vi "Curve Keypair.vi"(7 "path override":path, 8 "error in (no error)":errorcluster, 10 "z85_secret_key_":string, 11 "z85_public_key_":string) -> (0 "error out":errorcluster, 2 "z85_secret_key_ out":string, 3 "z85_public_key_ out":string)   [LabVIEW 2025, in "LibZMQ.lvlib"]
doc: "ZMQ_EXPORT int zmq_curve_keypair (char *z85_public_key_, char *z85_secret_key_);"
uses:
  LibZMQ.lvlib
  errno.vi
  strerror.vi
  <vilib>/Utility/error.llb/Error Cluster From Error Code.vi
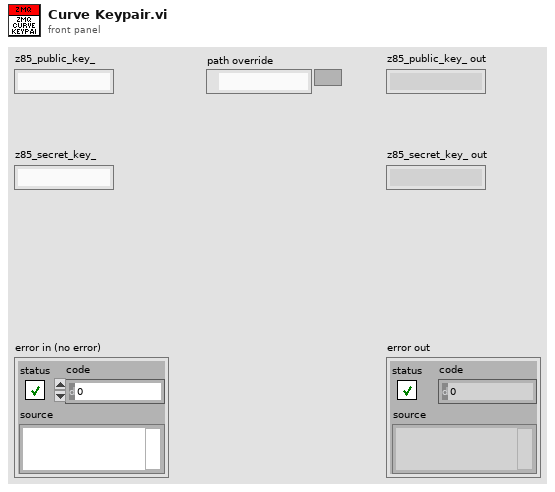
[diagram p1: front panel]
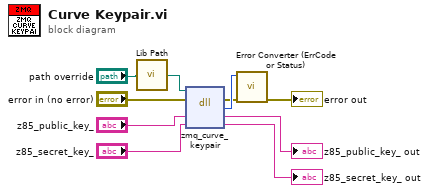
[diagram p0: block diagram]
diagram:
  n1 = call "Lib Path.vi"("path override"="path override") -> ("lib path"=w2:path)
  n2 = dll-call lib="C:/git/ZA/libzmq-v143-mt-4_3_6/lib/win32/libzmq-v143-mt-4_3_6.dll" fn="zmq_curve_keypair"(path in=w2, error in="error in (no error)", "z85_public_key_"="z85_public_key_", "z85_secret_key_"="z85_secret_key_") -> (error out=w4:errorcluster, "return type"=w10:i32, "z85_public_key_"=→"z85_public_key_ out":string, "z85_secret_key_"=→"z85_secret_key_ out":string)  [unwired: 1 in, 1 out]
  n3 = call "Error Converter (ErrCode or Status).vi"("error in (no error)"=w4, "error code"=w10) -> ("error out"=→"error out":errorcluster)  [unwired: 9 in]
